vi "Test_ImplicitlyNamedI32_ValueOK.vi"(8 "error in (no error)":errorcluster, 11 "TestCase in":refnum<class "TestCurrentValueTable.lvclass">) -> (0 "error out":errorcluster, 3 "TestCase out":refnum<class "TestCurrentValueTable.lvclass">)   [LabVIEW 2015, in "TestCurrentValueTable.lvclass"]
uses:
  TestCurrentValueTable.lvclass
  <vilib>/addons/_JKI Toolkits/VI Tester/TestCase.llb/TestCase.lvclass
  CurrentValueTable.lvclass
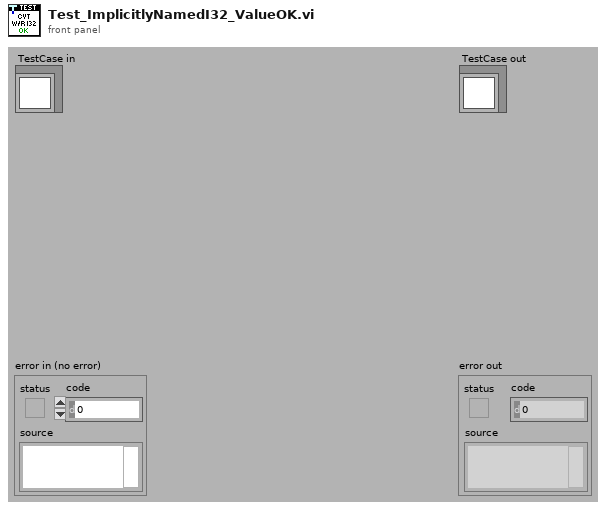
[diagram p1: front panel]
types:
  T1 = typedef "CurrentValueTable.lvlib/CurrentValueTable.lvclass/CurrentValueTable Reference.ctl" = refnum<data-value>
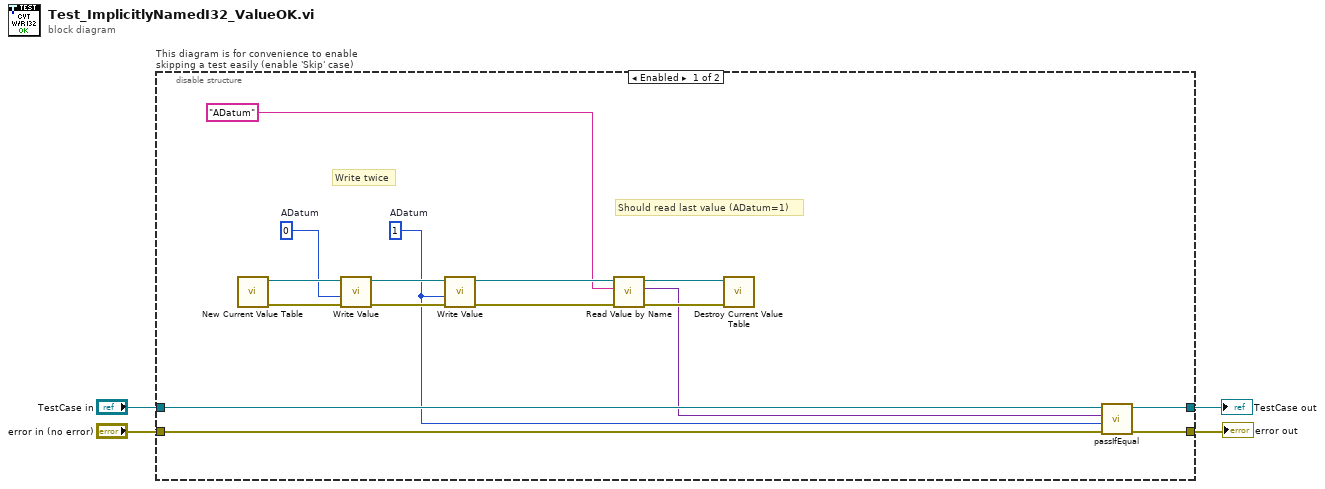
[diagram p0: block diagram]
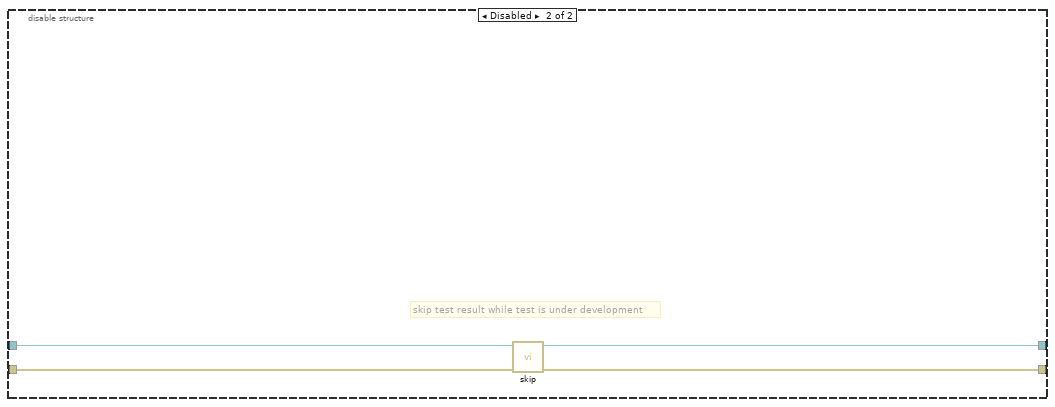
[diagram p2: hidden frame]
diagram:
  n1 = disable-structure "This diagram is for convenience to enable skipping a test easily (enable 'Skip' case)" shown="Enabled" {
    disable-tunnel: "TestCase in" -> [w20 w24]
    disable-tunnel: [w19 w22] -> w1
    disable-tunnel: [w18 w23] -> w3
    disable-tunnel: "error in (no error)" -> [w17 w21]
    frame Enabled {
      w5 = 1  # ADatum
      w6 = 0  # ADatum
      # "Write twice"
      # "Should read last value (ADatum=1)"
      n2 = call "New Current Value Table.vi"() -> ("error out"=w8:errorcluster, "Current Value Table"=w16:T1)  [unwired: 10 in]
      n3 = call "Write Value.vi"("error in (no error)"=w8, "Value"=w6, "Current Value Table"=w16) -> ("error out"=w7:errorcluster, "Current Value Table"=w9:T1)  [unwired: 7 in]
      n4 = call "Write Value.vi"("error in (no error)"=w7, "Value"=w5, "Current Value Table"=w9) -> ("error out"=w13:errorcluster, "Current Value Table"=w15:T1)  [unwired: 7 in]
      n5 = call "Read Value by Name.vi"("error in (no error)"=w13, "Data Name"="ADatum" ("Data Name (Use Value Name)"), "Current Value Table"=w15) -> ("error out"=w12:errorcluster, "Current Value"=w10:variant, "Current Value Table"=w14:T1)  [unwired: 5 in, 1 out]
      n6 = call "Destroy Current Value Table.vi"("error in (no error)"=w12, "Current Value Table"=w14) -> ()  [unwired: 9 in, 1 out]
      n7 = call-dynamic "passIfEqual.vi"("error in (no error)"=w17, "y"=w5, "x"=w10, "TestCase in"=w20) -> ("error out"=w18:errorcluster, "TestCase out"=w19:refnum<class "TestCurrentValueTable.lvclass">)  [unwired: 6 in]
    }
    frame Disabled {
      # "skip test result while test is under development"
      n8 = call <vilib>:"skip.vi"("error in (no error)"=w21, "TestCase in"=w24) -> ("error out"=w23:errorcluster, "TestCase out"=w22:refnum<class "TestCurrentValueTable.lvclass">)  [unwired: 8 in]
    }
  }
  "error out" <- w3
  "TestCase out" <- w1
